vi "ConsoleApplicationCall.vi"(6 "names":string[](array[string]), 7 "arguments name":string="args", 8 "error in":errorcluster, 11 "VI Interpreter in":refnum<class "VI Interpreter.lvclass">) -> (0 "error out":errorcluster, 3 "VI Interpreter out":refnum<class "VI Interpreter.lvclass">, 5 "Call":string)   [LabVIEW 2014, in "Raspberry Pi Compatible Compiler for LabVIEW.lvlib" / "PyConvBD.lvclass"]
uses:
  PyConvBD.lvclass
  VI Interpreter/Classes/VI Interpreter/VI Interpreter.lvclass
  Parsing/Python Functions.lvlib
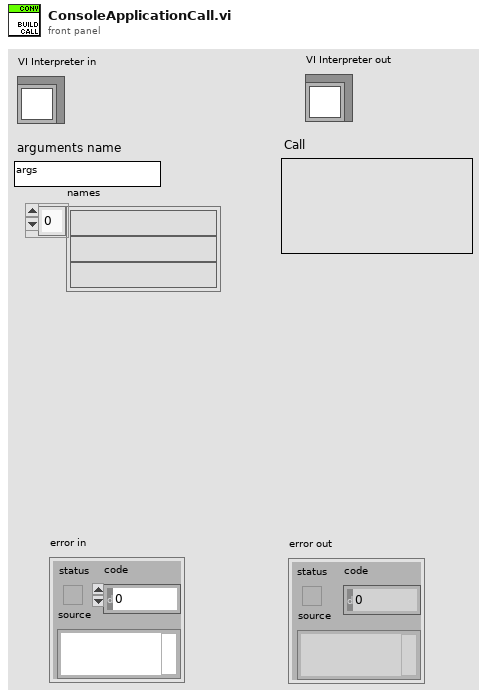
[diagram p1: front panel]
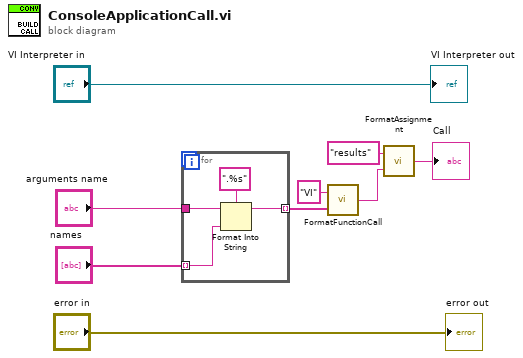
[diagram p0: block diagram]
diagram:
  n1 = for {
    tunnel: "arguments name" -> [w13]
    tunnel: "names" -> [w11] mode=indexing
    tunnel: [w10] -> w4 mode=indexing
    n2 = Format Into String(format string=".%s", initial string=w13, w11) -> (resulting string=w10:string)  [unwired: 1 in, 1 out]
  }
  n3 = call "FormatFunctionCall.vi"("parameters"=w4, "function"="VI") -> ("python object"=w2:string)
  n4 = call "FormatAssignment.vi"("value"=w2, "name"="results") -> ("python assignment"=→"Call":string)
  "error out" <- "error in"
  "VI Interpreter out" <- "VI Interpreter in"
